vi "VF_acumulo.vi"() -> ()   [LabVIEW 2018]
uses:
  <vilib>/measure/maspectr.llb/FFT Power Spectrum and PSD for 1 Chan (CDB).vi
  <vilib>/rtlsdr/rtlsdr.lvlib
  <vilib>/measure/NI_MAPro.lvlib
  <vilib>/Analysis/NI_AALPro.lvlib
panel:
  out "Integraded Spectrum":cluster{"f0":dbl, "df":dbl, "magnitude":dbl[]}[](graph)
  out "Frequencys":dbl[](array[numeric])
  out "F Count":i32
  out "size(s)":i32
  out "Power Spectrum 2":dbl[](graph)
  out "Power Spectrum":cluster{"f0":dbl, "df":dbl, "magnitude":dbl[]}[](graph)
  out "Center Frequency":dbl
  in  "config":bool
  in  "Number Of Samples":i32=16000
  in  "Center Frequency":u32=101000000
  in  "Sample Rate":u32=2400000
  out "function return":i32
  in  "Device Index":u32=1
  out "Device USB Strings":T1
  out "DeviceRefnum Out":u64
  in  "stop":bool
  out "Device Count":u32
  # "1"
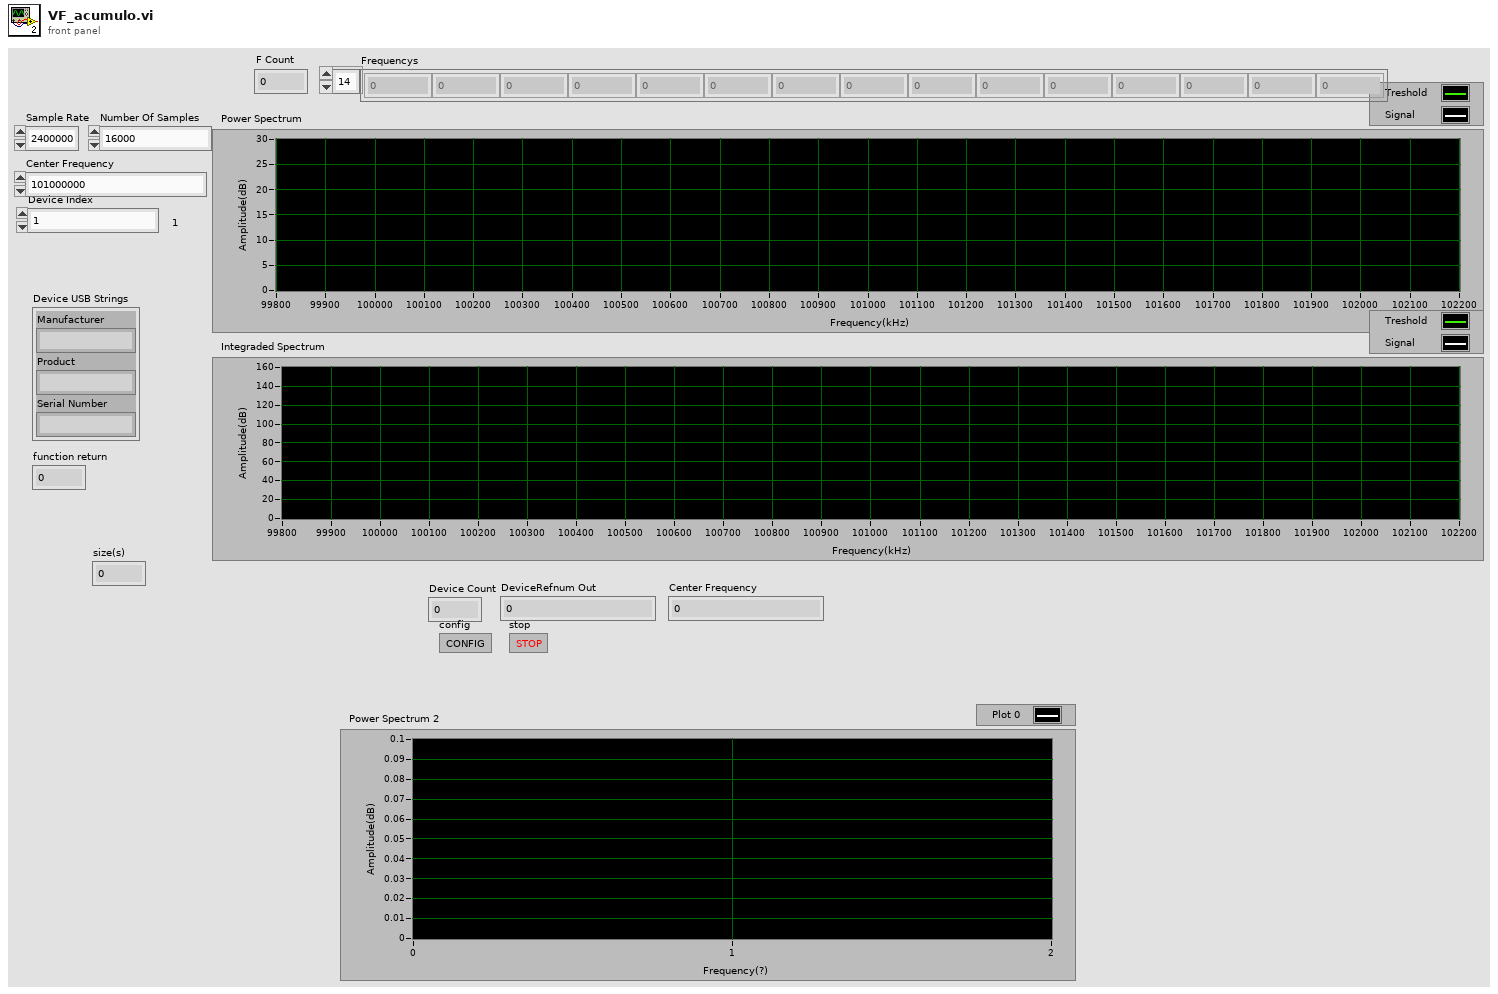
[diagram p1: front panel]
types:
  T1 = cluster{"Manufacturer":string, "Product":string, "Serial Number":string}
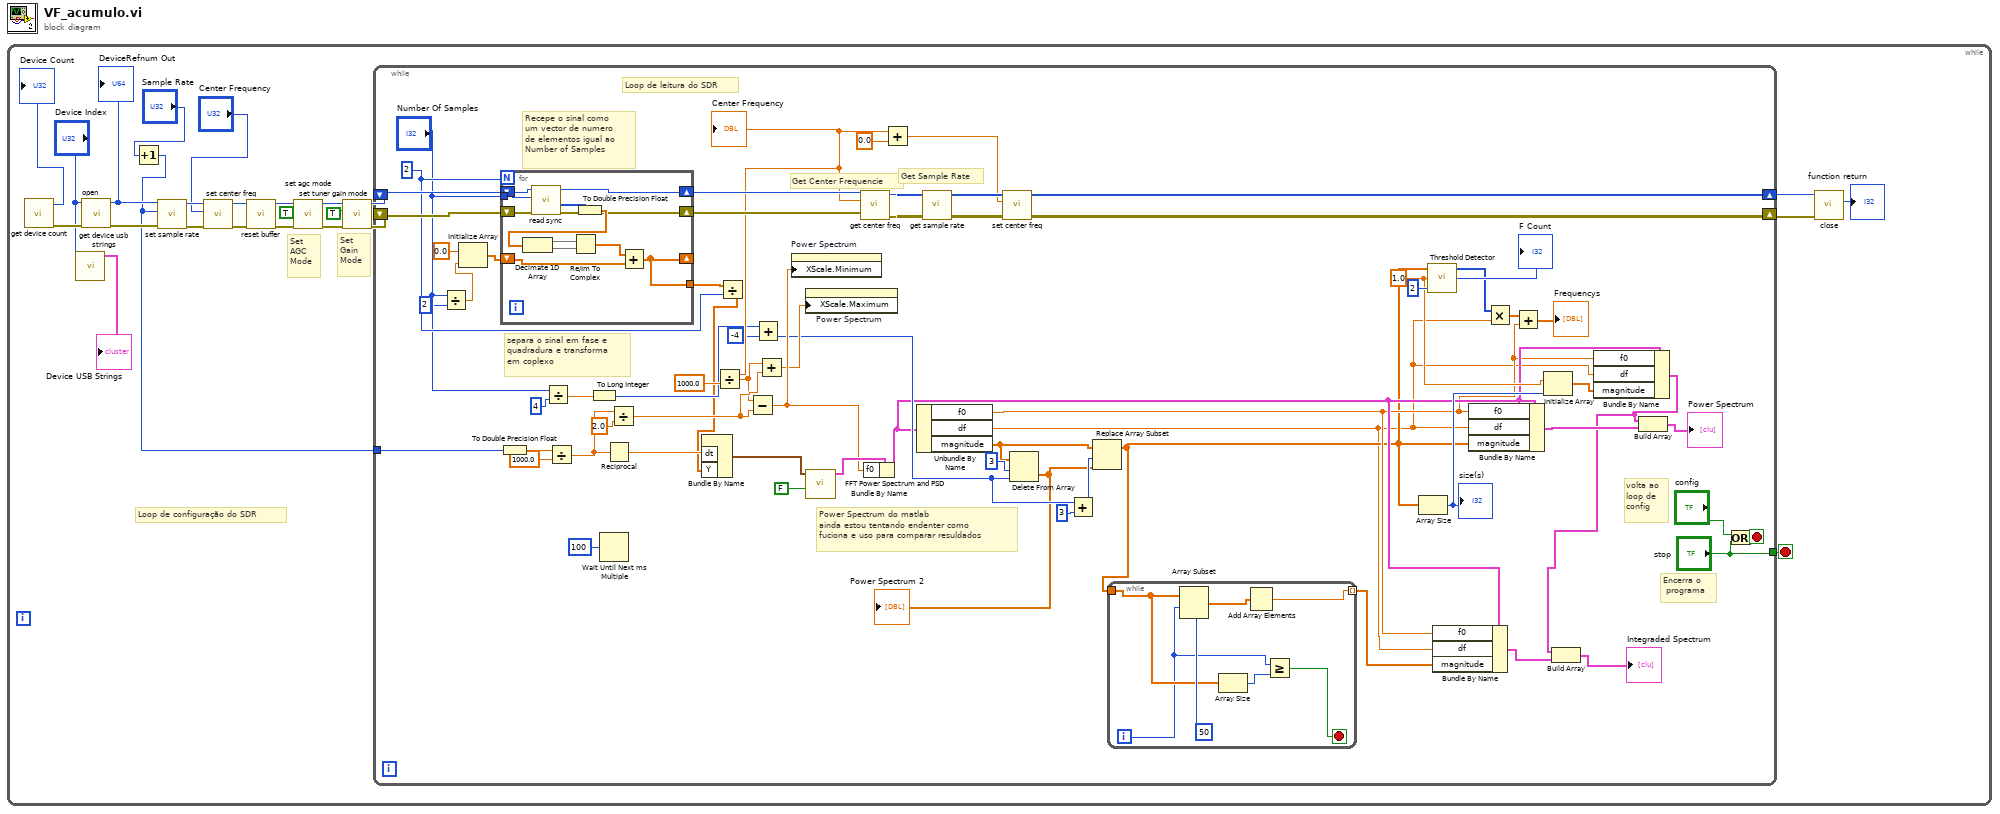
[diagram p0: block diagram]
diagram:
  n1 = while {
    stop <- w5 stop-if-true
    # "Set\nGain\nMode"
    # "Set\nAGC\nMode"
    # "Loop de configuração do SDR"
    n2 = call <vilib>:"get device count.vi"() -> ("error out"=w24:errorcluster, "Device Count"=→"Device Count":u32)  [unwired: 10 in]
    n3 = call <vilib>:"get device usb strings.vi"("Device Index"="Device Index") -> ("Device USB Strings"=→"Device USB Strings":T1)  [unwired: 8 in, 2 out]
    n4 = call <vilib>:"open.vi"("error in (no error)"=w24, "Device Index"="Device Index") -> ("error out"=w20:errorcluster, "DeviceRefnum Out"=w19:u64)  [unwired: 6 in]
    "DeviceRefnum Out" <- w19
    n5 = Increment(x="Sample Rate") -> (x+1=w1:u32)
    n6 = call <vilib>:"set sample rate.vi"("error in (no error)"=w20, "Sample Rate"=w1, "DeviceRefnum"=w19) -> ("error out"=w18:errorcluster, "DeviceRefnum Out"=w17:u64)  [unwired: 6 in, 1 out]
    n7 = call <vilib>:"set center freq.vi"("error in (no error)"=w18, "Center Frequency"="Center Frequency", "DeviceRefnum"=w17) -> ("error out"=w16:errorcluster, "DeviceRefnum Out"=w15:u64)  [unwired: 6 in, 1 out]
    n8 = call <vilib>:"reset buffer.vi"("error in (no error)"=w16, "DeviceRefnum"=w15) -> ("error out"=w14:errorcluster, "DeviceRefnum Out"=w13:u64)  [unwired: 7 in, 1 out]
    n9 = call <vilib>:"set agc mode.vi"("error in (no error)"=w14, "AGC Enable"=TRUE, "DeviceRefnum"=w13) -> ("error out"=w12:errorcluster, "DeviceRefnum Out"=w11:u64)  [unwired: 6 in, 1 out]
    n10 = call <vilib>:"set tuner gain mode.vi"("error in (no error)"=w12, "AutoGain"=TRUE ("AGC Enable"), "DeviceRefnum"=w11) -> ("error out"=w9:errorcluster, "DeviceRefnum Out"=w8:u64)  [unwired: 6 in, 1 out]
    n11 = while {
      shift-right: [w75] -> w6
      shift-left: w8 -> [w91]
      shift-right: [w74] -> w7
      shift-left: w9 -> [w92]
      tunnel: ["stop"] -> w5
      tunnel: w1 -> [w73]
      stop <- w89 stop-if-true
      w46 = 2
      w47 = 1.0 ("threshold")
      # "separa o sinal em fase e\nquadradura e transforma\nem coplexo"
      # "Recepe o sinal como\num vector de numero\nde elementos igual ao\nNumber of Samples"
      # "Encerra o\n programa"
      # "volta ao\nloop de \nconfig"
      # "Power Spectrum do matlab\nainda estou tentando endenter como \nfuciona e uso para comparar resuldados"
      # "Get Center Frequencie"
      # "Get Sample Rate"
      # "Loop de leitura do SDR"
      n12 = Divide(x="Number Of Samples", y=2) -> (x/y=w41:dbl)
      n13 = Initialize Array(0.0 ("element"), w41) -> (w43:dbl[])
      n14 = for {
        N: w46 -> [_]
        tunnel: "Number Of Samples" -> [w106]
        shift-right: [w105] -> w81
        shift-left: w92 -> [w111]
        shift-right: [w107] -> w86
        shift-left: w91 -> [w110]
        shift-right: [w101] -> _
        shift-left: w43 -> [w100]
        tunnel: [w101] -> w44
        n15 = call <vilib>:"read sync.vi"("error in (no error)"=w111, "Number Of Samples"=w106, "DeviceRefnum"=w110) -> ("error out"=w105:errorcluster, "Sample Buffer"=w108:u8[], "DeviceRefnum Out"=w107:u64)  [unwired: 5 in, 1 out]
        n16 = To Double Precision Float(number=w108) -> (double precision float=w109:dbl[])
        n17 = Decimate 1D Array(w109) -> (w104:dbl[], w103:dbl[])
        n18 = Re/Im To Complex(1:w103, 2:w104) -> (0:w102:cdb[])
        n19 = Add(x=w102, y=w100) -> (x+y=w101:cdb[])
      }
      n20 = To Double Precision Float(number=w73) -> (double precision float=w65:dbl)
      n21 = Divide(x="Number Of Samples", y=4) -> (x/y=w83:dbl)
      n22 = Divide(x=w65, y=1000.0) -> (x/y=w69:dbl)
      n23 = To Long Integer(number=w83) -> (32bit integer=w62:i32)
      n24 = Wait Until Next ms Multiple(millisecond multiple=u32 100) -> ()  [unwired: 1 out]
      n25 = Reciprocal(x=w69) -> (1/x=w71:dbl)
      n26 = Divide(x=w69, y=2.0) -> (x/y=w59:dbl)
      n27 = Divide(x=w44, y=w46) -> (x/y=w45:cdb[])
      n28 = Bundle By Name("dt"=w71, "Y"=w45) -> (w72:waveform(cdb))  [unwired: 1 in]
      n29 = Add(x=w62, y=-4) -> (x+y=w36:i32)
      n30 = call-poly <vilib>:"FFT Power Spectrum and PSD.vi"("dB On (F)"=FALSE, "time signal"=w72) -> ("Power Spectrum / PSD"=w64:cluster{"f0":dbl, "df":dbl, "magnitude":dbl[]})  [unwired: 6 in, 3 out]
      n31 = call <vilib>:"get center freq.vi"("error in (no error)"=w81, "DeviceRefnum"=w86) -> ("error out"=w80:errorcluster, "Center Frequency"=w67:dbl, "DeviceRefnum Out"=w82:u64)  [unwired: 7 in]
      "Center Frequency" <- w67
      n32 = Divide(x=w67, y=1000.0) -> (x/y=w58:dbl)
      n33 = Subtract(x=w58, y=w59) -> (x-y=w60:dbl)
      n34 = Add(x=w58, y=w59) -> (x+y=w57:dbl)
      n35 = property on="Power Spectrum" class="WFGraph (strict)"("XScale.Minimum"=w60) -> ()  [unwired: 2 in, 2 out]
      n36 = property on="Power Spectrum" class="WFGraph (strict)"("XScale.Maximum"=w57) -> ()  [unwired: 2 in, 2 out]
      n37 = Bundle By Name(cluster=w64, "f0"=w60) -> (w33:cluster{"f0":dbl, "df":dbl, "magnitude":dbl[]})
      n38 = Add(x=w67, y=0.0) -> (x+y=w76:dbl)
      n39 = Unbundle By Name(w33) -> ("f0"=w32:dbl, "df"=w27:dbl, "magnitude"=w38:dbl[])
      n40 = call <vilib>:"get sample rate.vi"("error in (no error)"=w80, "DeviceRefnum"=w82) -> ("error out"=w79:errorcluster, "DeviceRefnum Out"=w78:u64)  [unwired: 7 in, 1 out]
      n41 = call <vilib>:"set center freq.vi"("error in (no error)"=w79, "Center Frequency"=w76, "DeviceRefnum"=w78) -> ("error out"=w74:errorcluster, "DeviceRefnum Out"=w75:u64)  [unwired: 6 in, 1 out]
      n42 = Delete From Array(array=w38, length=3, index=w36) -> (deleted portion=w34:dbl[])  [unwired: 1 out]
      "Power Spectrum 2" <- w34
      n43 = Add(x=w36, y=3) -> (x+y=w37:i32)
      n44 = Replace Array Subset(array=w38, new element=w34, index=w37) -> (w28:dbl[])
      n45 = while {
        tunnel: w28 -> [w95]
        tunnel: [w98] -> w26 mode=indexing
        i -> [w94]
        stop <- w93 stop-if-true
        n46 = Array Subset(array=w95, index=w94, length=50) -> (w99:dbl[])
        n47 = Array Size(array=w95) -> (size(s)=w96:i32)
        n48 = Add Array Elements(numeric array=w99) -> (sum=w98:dbl)
        n49 = Greater Or Equal?(x=w94, y=w96) -> (x >= y?=w93:bool)
      }
      n50 = Array Size(array=w28) -> (size(s)=w50:i32)
      "size(s)" <- w50
      n51 = call <vilib>:"Threshold Detector.vi"("width"=2, "threshold"=w47, "X"=w28) -> ("count"=→"F Count":i32, "Indices"=w55:i32[])  [unwired: 1 out]
      n52 = Bundle By Name(cluster=w33, "f0"=w32, "df"=w27, "magnitude"=w26) -> (w30:cluster{"f0":dbl, "df":dbl, "magnitude":dbl[]})
      n53 = Bundle By Name(cluster=w33, "f0"=w32, "df"=w27, "magnitude"=w28) -> (w52:cluster{"f0":dbl, "df":dbl, "magnitude":dbl[]})
      n54 = Multiply(x=w55, y=w27) -> (x*y=w54:dbl[])
      n55 = Add(x=w54, y=w32) -> (x+y=→"Frequencys":dbl[])
      n56 = Initialize Array(w47, w50) -> (w49:dbl[])
      n57 = Bundle By Name(cluster=w33, "f0"=w32, "df"=w27, "magnitude"=w49) -> (w31:cluster{"f0":dbl, "df":dbl, "magnitude":dbl[]})
      n58 = Build Array(w31, w30) -> (→"Integraded Spectrum":cluster{"f0":dbl, "df":dbl, "magnitude":dbl[]}[])
      n59 = Build Array(w31, w52) -> (→"Power Spectrum":cluster{"f0":dbl, "df":dbl, "magnitude":dbl[]}[])
      n60 = Or(x="config", y="stop") -> (x .or. y?=w89:bool)
    }
    n61 = call <vilib>:"close.vi"("error in (no error)"=w7, "DeviceRefnum"=w6) -> ("function return"=→"function return":i32)  [unwired: 8 in, 1 out]
  }
